vi "Destroy.vi"(8 "error in (no error)":errorcluster, 11 "Plugin Manager in":refnum<class "CIFPluginManager.lvclass">) -> (0 "error out":errorcluster, 3 "Plugin Manager out":refnum<class "CIFPluginManager.lvclass">)   [LabVIEW 2021, in "CIFPluginManager.lvclass"]
uses:
  CIFPluginManager.lvclass
  CIFPluginManager.lvclass/CIFPluginManager.ctl
  <vilib>/gRPC/LabVIEW gRPC Servicer/ServiceBase/ServiceBase.lvclass
  typedef/Trigger Discovery User Event.ctl
  CIFCore/Common/Typedef/Version.ctl
  CIFCore/Common/CIFCoreCommon.lvlib
  typedef/Plugin Metadata.ctl
  typedef/Discovered Plugin.ctl
  typedef/Discovery User Event.ctl
  typedef/Discovery Events.ctl
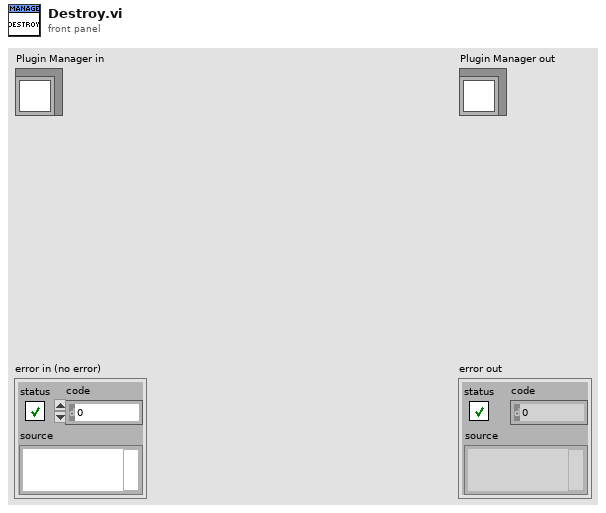
[diagram p1: front panel]
types:
  T1 = typedef "CIFPluginManager.lvclass/Discovery Events.ctl" = cluster{"Trigger Discovery":T2, "Discovery":T3, "Shutdown":refnum<user-event>}
  T2 = typedef "CIFPluginManager.lvclass/Trigger Discovery User Event.ctl" = refnum<user-event>
  T3 = typedef "CIFPluginManager.lvclass/Discovery User Event.ctl" = refnum<user-event>
  T4 = typedef "CIFPluginManager.lvclass/Plugin Management Data.ctl" = cluster{"vi reference":refnum<vi>, "gRPC ID":T5, "Plugin Type":string, "Unique Name":string, "gRPC Port":i32, "Version":T6, "Load Timestamp":i64, "Unload Timestamp":i64, "Unloading":bool, "Ready for removal":bool, "status":T7}
  T5 = typedef "grpc-lvsupport-release.lvlib/grpcId.ctl" = u64
  T6 = typedef "CIFCoreCommon.lvlib/Version.ctl" = cluster{"Major":i32, "Minor":i32, "Fix":i32, "Build":i32}
  T7 = typedef "CIF_Manager_server.lvlib/cif_plugincore_StatusData.ctl" = cluster{"state":T8, "timing_statistics":T9, "fifo_statistics":T11, "error":T12, "monitor_doubles":T13, "monitor_u64s":T14, "monitor_i64s":T15}
  T8 = typedef "CIF_Manager_server.lvlib/cif_plugincore_StatusData_State.ctl" = enum32{"NULL", "CREATING", "LISTENING", "RUNNING", "CLEANINGUP", "DESTROYING"}
  T9 = typedef "CIF_Manager_server.lvlib/cif_plugincore_TimingStatistics.ctl" = cluster{"period":T10, "wake_error":T10, "execute":T10, "housekeep":T10, "idle":T10, "cleanup":T10, "custom_1":T10, "custom_2":T10}
  T10 = typedef "CIF_Manager_server.lvlib/cif_common_TimingStats.ctl" = cluster{"max":i64, "min":i64, "avg":dbl}
  T11 = typedef "CIF_Manager_server.lvlib/cif_plugincore_FifoStatistics.ctl" = cluster{"from_t0":T10, "from_previous_plugin":T10, "output_error":T10}
  T12 = typedef "CIF_Manager_server.lvlib/cif_plugincore_Error.ctl" = cluster{"status":bool, "code":i32}
  T13 = typedef "CIF_Manager_server.lvlib/cif_plugincore_MonitorDoubles.ctl" = cluster{"double_1":dbl, "double_2":dbl, "double_3":dbl, "double_4":dbl}
  T14 = typedef "CIF_Manager_server.lvlib/cif_plugincore_MonitorU64.ctl" = cluster{"u64_1":u64, "u64_2":u64, "u64_3":u64, "u64_4":u64}
  T15 = typedef "CIF_Manager_server.lvlib/cif_plugincore_MonitorI64.ctl" = cluster{"i64_1":i64, "i64_2":i64, "i64_3":i64, "i64_4":i64}
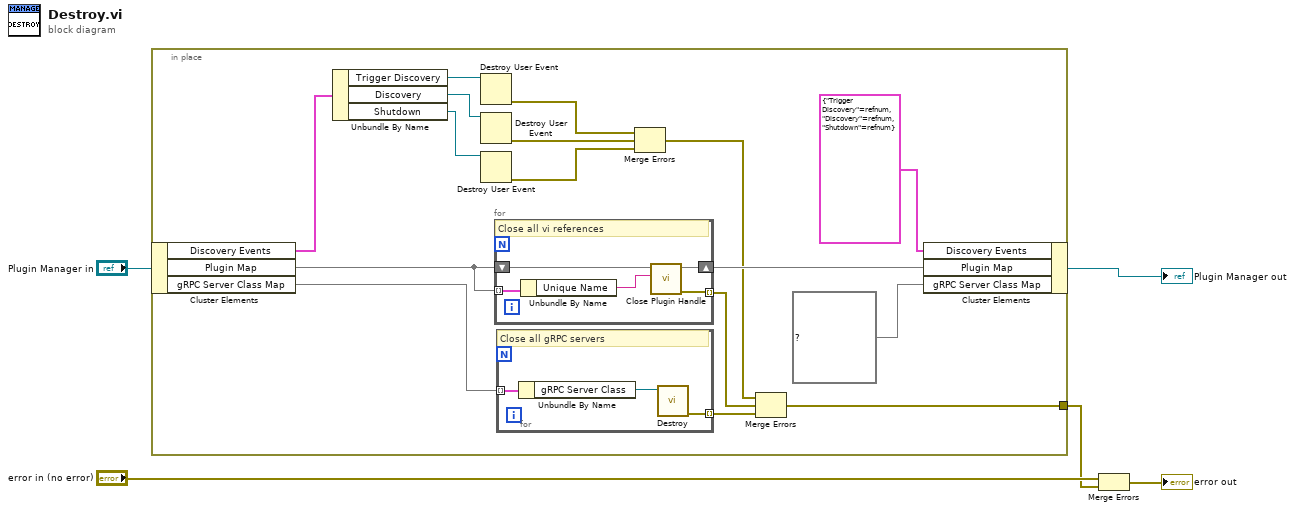
[diagram p0: block diagram]
diagram:
  n1 = in-place {
    in-place-border: [w18] -> w1
    n2 = in-place-cluster #1("Plugin Manager in") -> ("Discovery Events"=w13:T1, "Plugin Map"=w16:map{string, T4}, "gRPC Server Class Map"=w21:map{string, refnum<class "ServiceBase.lvclass">})
    n3 = Unbundle By Name(w13) -> ("Trigger Discovery"=w12:T2, "Discovery"=w10:T3, "Shutdown"=w11:refnum<user-event>)
    n4 = Destroy User Event(user event=w12) -> (error out=w7:errorcluster)  [unwired: 1 in]
    n5 = Destroy User Event(user event=w10) -> (error out=w8:errorcluster)  [unwired: 1 in]
    n6 = Destroy User Event(user event=w11) -> (error out=w9:errorcluster)  [unwired: 1 in]
    n7 = for {
      tunnel: w16 -> [w26] mode=indexing
      shift-right: [w23] -> w15
      shift-left: w16 -> [w25]
      tunnel: [w22] -> w17 mode=indexing
      # "Close all vi references"
      n8 = Unbundle By Name(w26) -> ("Unique Name"=w24:string)
      n9 = call "Close Plugin Handle.vi"("Unique Name"=w24, "Plugin Map in"=w25) -> ("error out"=w22:errorcluster, "Plugin Map out"=w23:map{string, T4})  [unwired: 8 in]
    }
    n10 = for {
      tunnel: w21 -> [w29] mode=indexing
      tunnel: [w27] -> w19 mode=indexing
      # "Close all gRPC servers"
      n11 = Unbundle By Name(w29) -> ("gRPC Server Class"=w28:refnum<class "ServiceBase.lvclass">)
      n12 = call-dynamic "Destroy.vi"("SignalGeneratorService in"=w28) -> ("error out"=w27:errorcluster)  [unwired: 9 in, 1 out]
    }
    n13 = Merge Errors(w7, w8, w9) -> (w6:errorcluster)
    n14 = Merge Errors(w6, w17, w19) -> (w18:errorcluster)
    n15 = in-place-cluster #1("Discovery Events"=T1 {"Trigger Discovery"=refnum, "Discovery"=refnum, "Shutdown"=refnum}, "Plugin Map"=w15, "gRPC Server Class Map"=map{string, refnum<class "ServiceBase.lvclass">} {}) -> (→"Plugin Manager out":refnum<class "CIFPluginManager.lvclass">)
  }
  n16 = Merge Errors("error in (no error)", w1) -> (→"error out":errorcluster)
